vi "Sleep For.vi"   [LabVIEW 2013, in "Linux RT Utilities.lvlib"]
doc: "This VI sleeps the calling thread for the specified relative time."
uses:
  Linux RT Utilities.lvlib
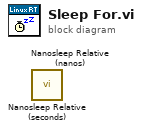
[diagram p0: block diagram]
diagram:
  n1 = call "Nanosleep Relative (seconds).vi"() -> ()  [unwired: 11 in, 1 out]
  n2 = call "Nanosleep Relative (nanos).vi"() -> ()  [unwired: 11 in, 1 out]
